vi "ExtendedTimer FGV.vi"(8 "error in":errorcluster, 10 "Timeout (s)":dbl=5.0, 11 "Timer Action":T1) -> (0 "error out":errorcluster, 2 "Done?":bool, 3 "Elapsed Time":dbl)   [LabVIEW 2024]
doc: "This functional global is used to keep track of the elapsed time in a given sequence step."
uses:
  TypeDefs/ExtendedTimer Actions.ctl
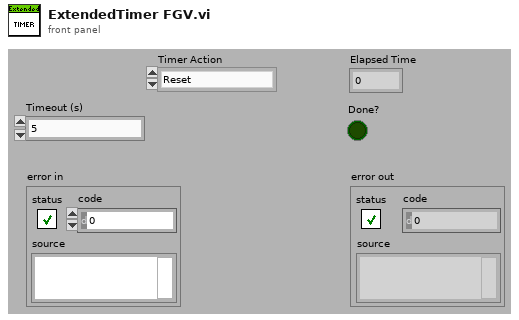
[diagram p1: front panel]
types:
  T1 = typedef "ExtendedTimer Actions.ctl" = enum16{"Reset", "Check Time", "Pause", "Resume", "SetTimeOut"}
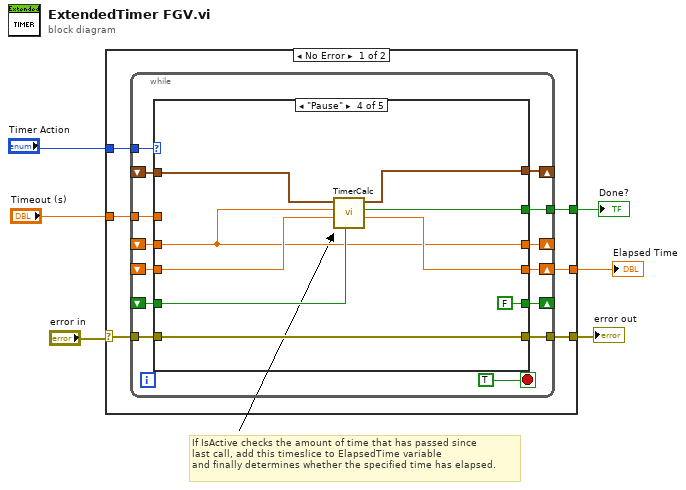
[diagram p0: block diagram]
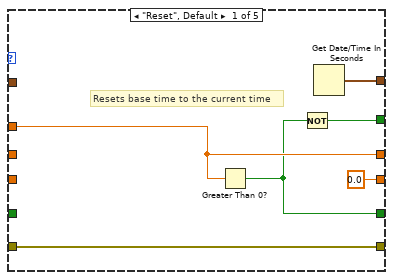
[diagram p2: hidden frame]
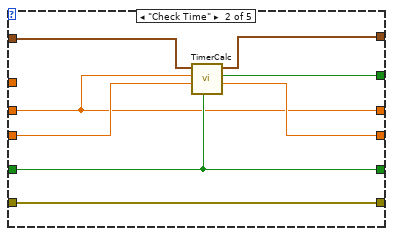
[diagram p3: hidden frame]
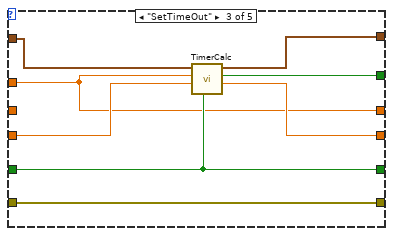
[diagram p4: hidden frame]
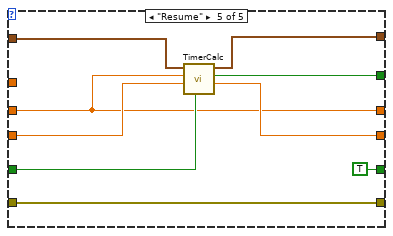
[diagram p5: hidden frame]
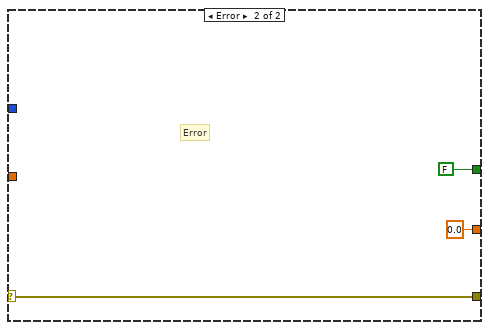
[diagram p6: hidden frame]
diagram:
  # "If IsActive checks the amount of time that has passed since\nlast call, add this timeslice to ElapsedTime variable \nand finally determines whether the specified time has elapsed."
  n1 = case shown="No Error" "error in" {
    selector: "error in" -> [w12 w69]
    tunnel: [w7 w69] -> w5
    tunnel: "Timer Action" -> [w11 _]
    tunnel: "Timeout (s)" -> [w10 _]
    tunnel: [w9 0.0] -> w3
    tunnel: [w8 FALSE] -> w2
    frame No Error {
      n2 = while {
        tunnel: w12 -> [w18]
        tunnel: w11 -> [w25]
        tunnel: w10 -> [w24]
        shift-right: [w23] -> _
        shift-left: _ -> [w20]
        tunnel: [w21] -> w8
        tunnel: [w19] -> w7
        shift-right: [w17] -> _
        shift-left: _ -> [w15]
        shift-right: [w22] -> w9
        shift-left: _ -> [w16]
        shift-right: [w14] -> _
        shift-left: _ -> [w13]
        stop <- TRUE stop-if-true
        n3 = case shown="\"Pause\"" w25 {
          tunnel: w24 -> [w29 _ w41 _ _]
          tunnel: [w32 w34 w42 w49 w58] -> w23
          tunnel: [0.0 w36 w44 w53 w62] -> w22
          tunnel: [w27 w38 w46 w51 w61] -> w21
          tunnel: w20 -> [_ w40 w48 w55 w64]
          tunnel: [w30 w39 w47 w56 w65] -> w19
          tunnel: w18 -> [w30 w39 w47 w56 w65]
          tunnel: [w28 w37 w45 FALSE TRUE] -> w17
          tunnel: w16 -> [_ w35 w43 w54 w63]
          tunnel: w15 -> [_ w37 w45 w52 w60]
          tunnel: [w29 w33 w41 w50 w59] -> w14
          tunnel: w13 -> [_ w33 _ w50 w59]
          frame "Reset", Default {
            # "Resets base time to the current time"
            n4 = Greater Than 0?(x=w29) -> (x > 0?=w28:bool)
            n5 = Not(x=w28) -> (.not. x?=w27:bool)
            n6 = Get Date/Time In Seconds() -> (seconds since 1Jan1904=w32:timestamp)
          }
          frame "Check Time" {
            n7 = call "TimerCalc.vi"("Active"=w37, "ElapsedTime in"=w35, "Timeout[s]"=w33, "timeOfLastCall"=w40) -> ("ElapsedTime out"=w36:dbl, "Done"=w38:bool, "now"=w34:timestamp)  [unwired: 5 in]
          }
          frame "SetTimeOut" {
            n8 = call "TimerCalc.vi"("Active"=w45, "ElapsedTime in"=w43, "Timeout[s]"=w41, "timeOfLastCall"=w48) -> ("ElapsedTime out"=w44:dbl, "Done"=w46:bool, "now"=w42:timestamp)  [unwired: 5 in]
          }
          frame "Pause" {
            n9 = call "TimerCalc.vi"("Active"=w52, "ElapsedTime in"=w54, "Timeout[s]"=w50, "timeOfLastCall"=w55) -> ("ElapsedTime out"=w53:dbl, "Done"=w51:bool, "now"=w49:timestamp)  [unwired: 5 in]
          }
          frame "Resume" {
            n10 = call "TimerCalc.vi"("Active"=w60, "ElapsedTime in"=w63, "Timeout[s]"=w59, "timeOfLastCall"=w64) -> ("ElapsedTime out"=w62:dbl, "Done"=w61:bool, "now"=w58:timestamp)  [unwired: 5 in]
          }
        }
      }
    }
    frame Error {
      # "Error"
    }
  }
  "error out" <- w5
  "Elapsed Time" <- w3
  "Done?" <- w2
